vi "Control Panel.vi"(8 "error in (no error)":errorcluster, 11 "Power Supply.lvclass":refnum<class "Power Supply.lvclass">) -> (0 "error out":errorcluster, 3 "Power Supply.lvclass out":refnum<class "Power Supply.lvclass">)   [LabVIEW 2017, in "Power Supply.lvclass"]
uses:
  Power Supply.lvclass
  Utility Classes/InstrPtr/InstrPtr.lvclass
  Magnet status.ctl
  Power Supply.lvclass/Power Supply.ctl
  Global/Relative Sound Files.vi
  File IO/File IO.lvclass
panel:
  out "Was at persistent?":bool
  in  "Return to persistent?":bool
  out "log counter":dbl
  out "Going to Field?":bool
  out "Current Field":dbl[unit]
  out "Update UI":bool
  out "Status":T1
  out "*ips120":T2
  in  "Abort Field Sweep":bool
  out "done?":bool
  out "ILM Shut Down?":bool
  out "SH On":bool caption="Switch Heater"
  out "Persistent Mode":bool
  in  "SHcontrol":bool caption="Switch Heater"
  in  "gotopersistent":bool
  out "active":bool
  in  "Train\nMagnet":bool
  out "Busy":bool
  out "ready?":bool
  in  "rate":dbl[unit]=0.016666666666666666 caption="Rate" min=0.0 max=0.25
  in  "Goto":dbl[unit]
  in  "Clamp":bool
  in  "Check for Magnet":bool
  in  "Hold":bool
  in  "Goto Zero":bool
  in  "Goto Field":bool
  in  "endprgm":bool
  # "Magnet Control Panel"
  # "(at current field)"
  # "Off"
  # "On"
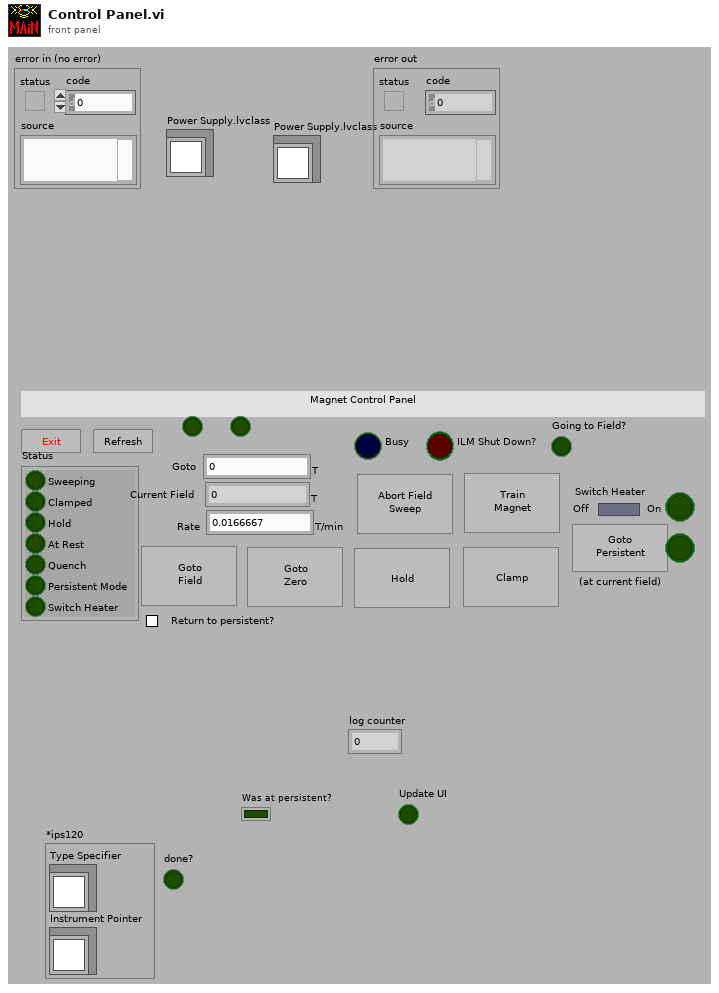
[diagram p1: front panel]
types:
  T1 = typedef "Power Supply.lvclass/Magnet status.ctl" = cluster{"Sweeping":bool, "Clamped":bool, "Hold":bool, "At Rest":bool, "Quench":bool, "Persistent Mode":bool, "Switch Heater":bool}
  T2 = cluster{"Type Specifier":refnum<class "Power Supply.lvclass">, "Instrument Pointer":refnum<class "InstrPtr.lvclass">}
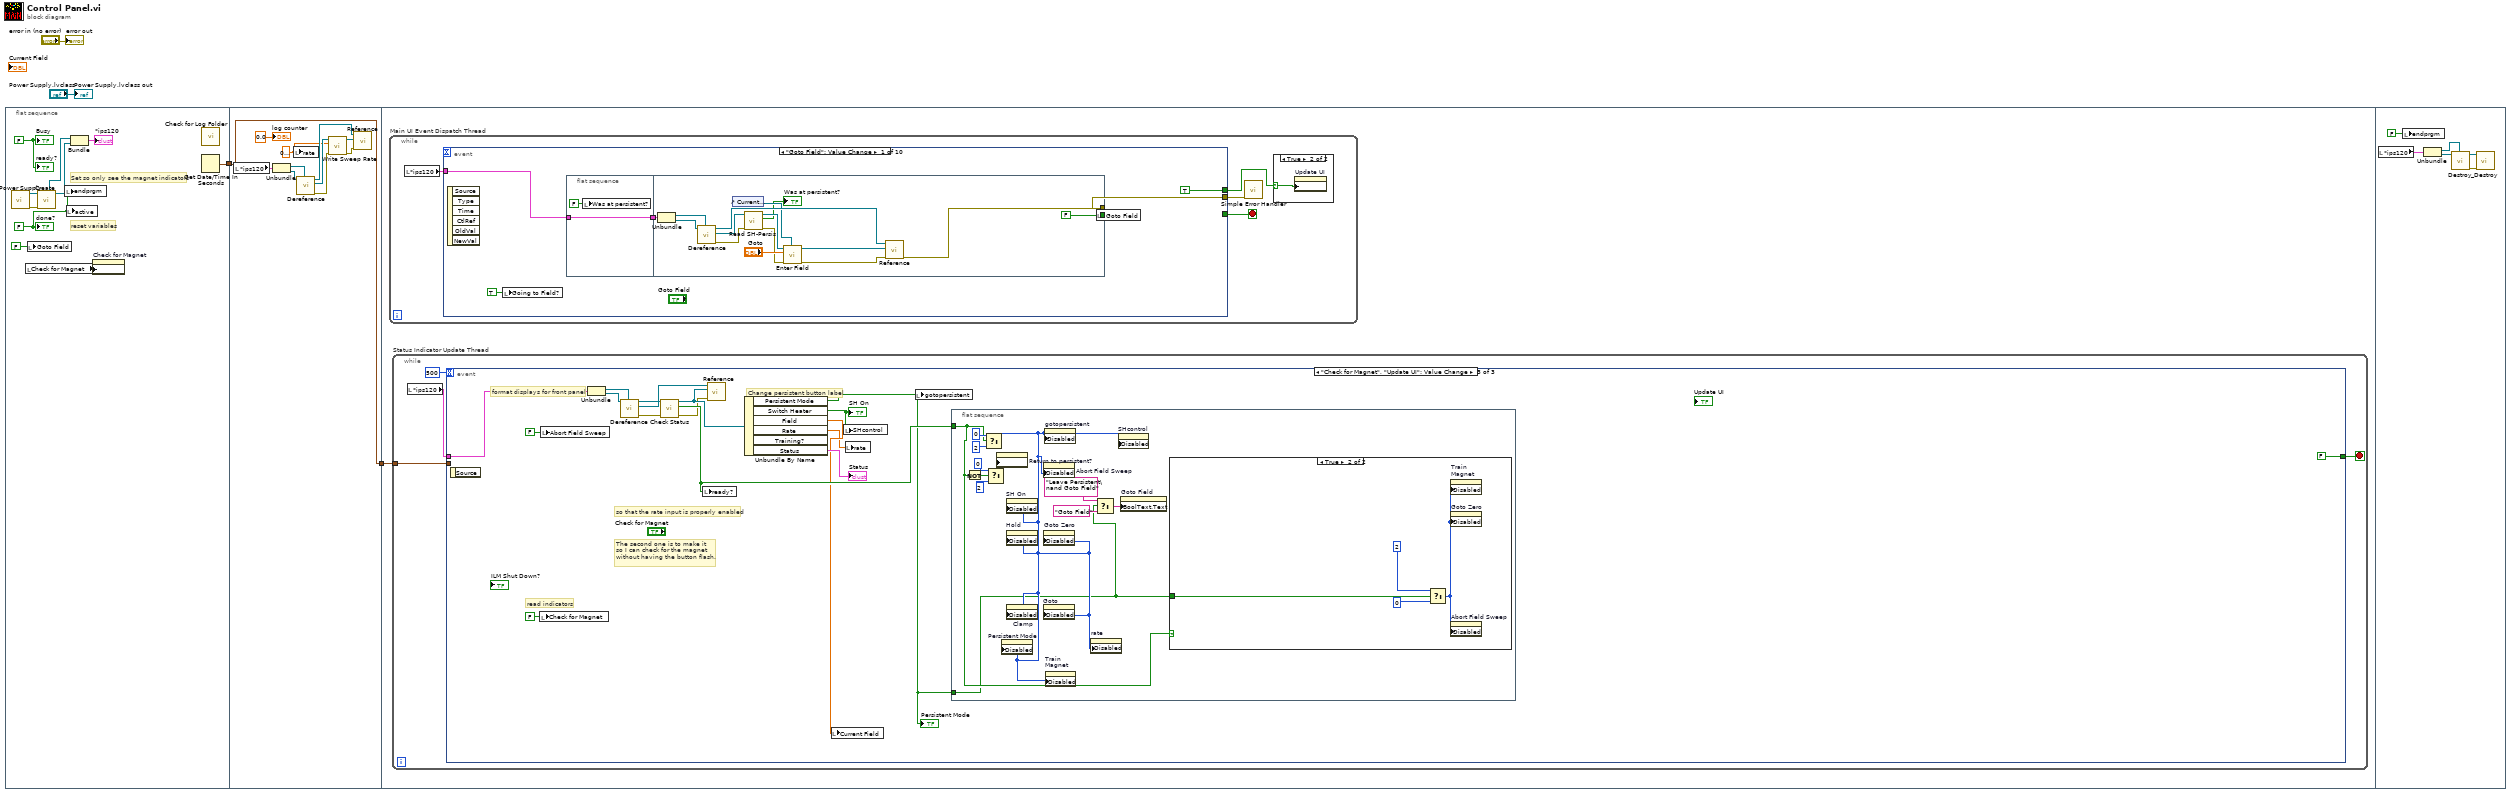
[diagram p0: block diagram]
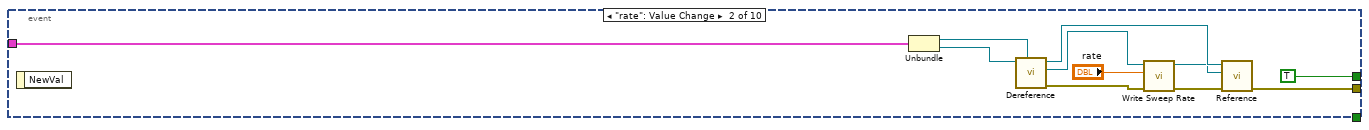
[diagram p3: hidden frame]
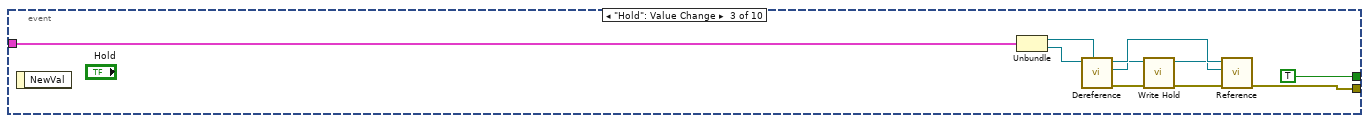
[diagram p4: hidden frame]
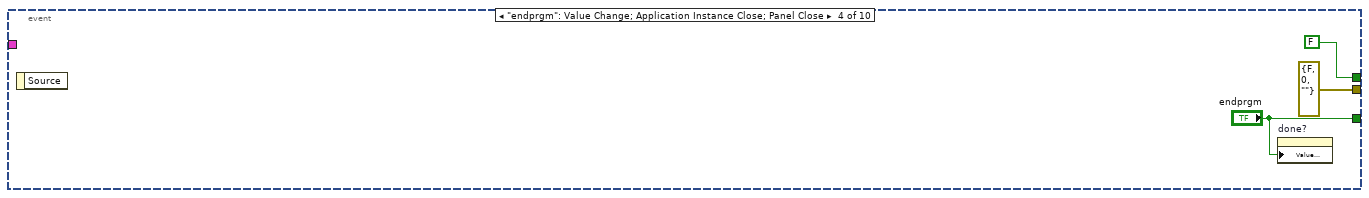
[diagram p5: hidden frame]
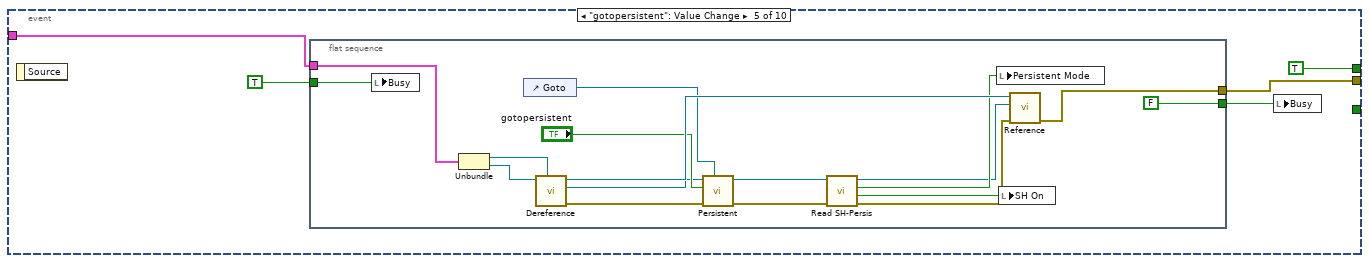
[diagram p6: hidden frame]
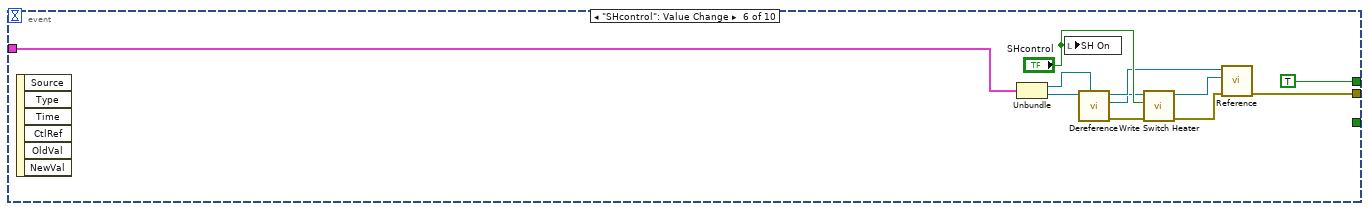
[diagram p7: hidden frame]
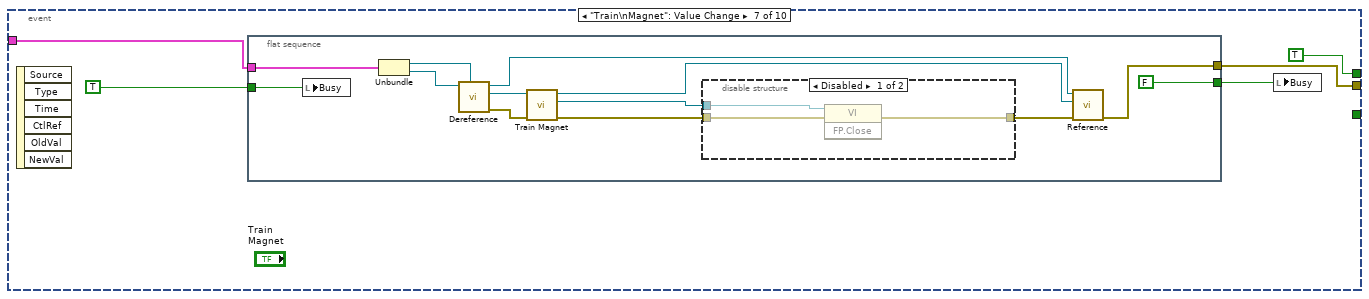
[diagram p8: hidden frame]
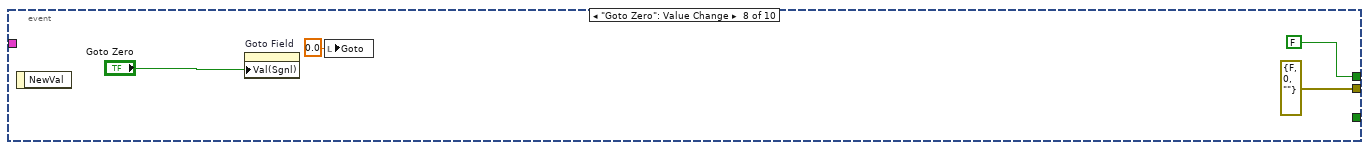
[diagram p10: hidden frame]
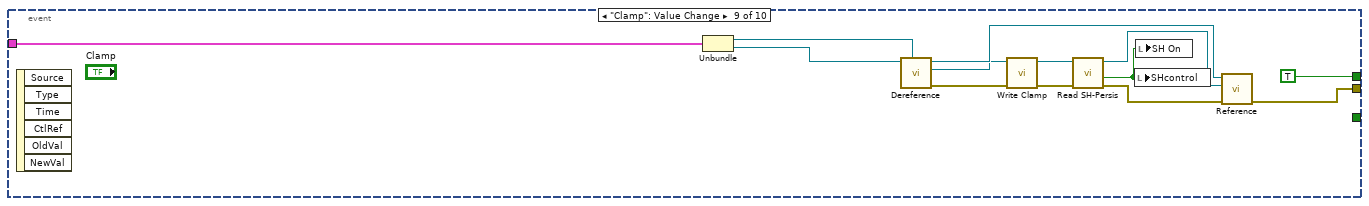
[diagram p11: hidden frame]
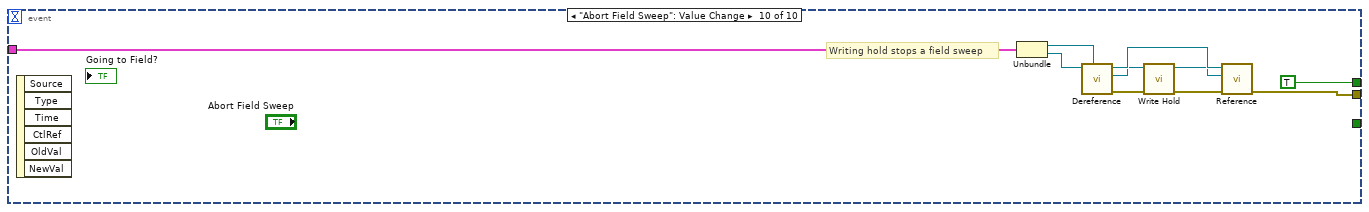
[diagram p12: hidden frame]
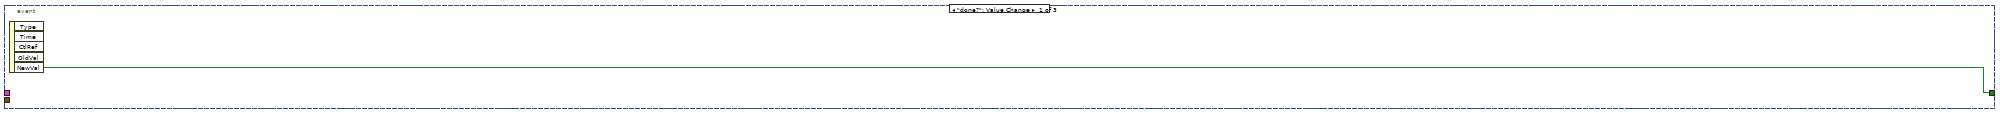
[diagram p13: hidden frame]
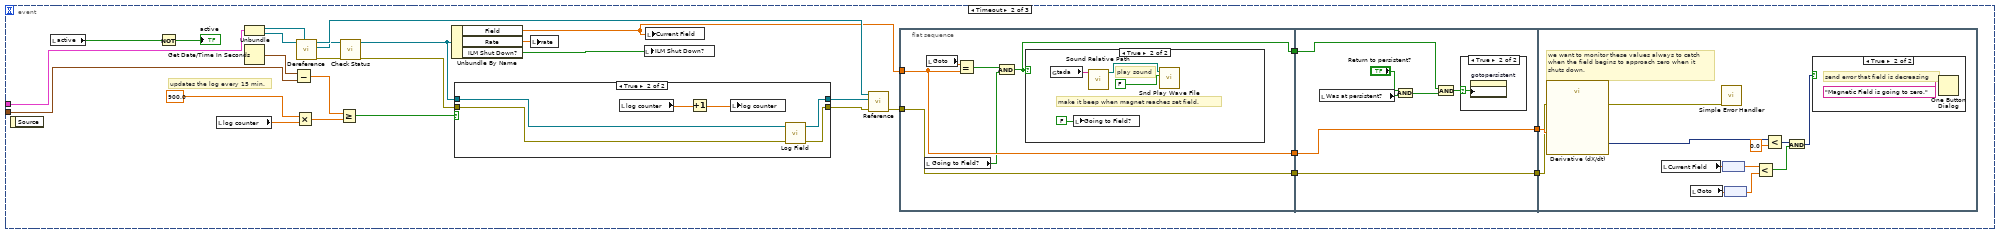
[diagram p14: hidden frame]
diagram:
  n1 = flat-sequence {
    tunnel: [w5] -> w2
    tunnel: w2 -> [w16]
    tunnel: [w16] -> w1
    tunnel: w1 -> [w26]
    frame #0 {
      w14 = FALSE
      w12 = FALSE
      # "Set so only see the magnet indicators"
      # "reset variables"
      n2 = call "Power Supply.vi"() -> ("error out"=w7:errorcluster, "Power Supply out"=w11:refnum<class "Power Supply.lvclass">)  [unwired: 10 in]
      n3 = local read "Check for Magnet"() -> (w13:bool)
      n4 = local write "Goto Field"(FALSE ("active")) -> ()
      n5 = call "Create.vi"("error in (no error)"=w7, "Instrument in"=w11) -> ("Instrument Pointer"=w10:refnum<class "InstrPtr.lvclass">, "Type Specifier"=w9:refnum<class "Power Supply.lvclass">)  [unwired: 7 in, 1 out]
      n6 = local write "endprgm"(w12) -> ()
      n7 = local write "active"(w12) -> ()
      n8 = Bundle("Type Specifier"=w9, "Instrument Pointer"=w10) -> (→"*ips120":T2)  [unwired: 1 in]
      n9 = property on="Check for Magnet" class="Bool (strict)"("Value (Signaling)"=w13) -> ()  [unwired: 2 in, 2 out]
      n10 = call "Check for Log Folder.vi"() -> ()  [unwired: 1 out]
      n11 = Get Date/Time In Seconds() -> (seconds since 1Jan1904=w5:timestamp)
      "ready?" <- w14
      "Busy" <- w14
      "done?" <- w12
    }
    frame #1 {
      w17 = dbl[unit] 0.016666666666666666 ("rate")
      n12 = local read "*ips120"() -> (w18:T2)
      n13 = Unbundle(w18) -> ("Type Specifier"=w19:refnum<class "Power Supply.lvclass">, "Instrument Pointer"=w20:refnum<class "InstrPtr.lvclass">)
      n14 = local write "rate"(w17) -> ()
      n15 = call "Dereference.vi"("Type Specifier"=w19, "InstrPtr"=w20) -> ("error out"=w24:errorcluster, "Instrument out"=w23:refnum<class "Power Supply.lvclass">, "InstrPtr out"=w21:refnum<class "InstrPtr.lvclass">)  [unwired: 7 in]
      n16 = call-dynamic "Write Sweep Rate.vi"("error in (no error)"=w24, "rate"=w17, "Power Supply in"=w23) -> ("error out"=w25:errorcluster, "Power Supply out"=w22:refnum<class "Power Supply.lvclass">)  [unwired: 7 in]
      n17 = call "Reference.vi"("error in (no error)"=w25, "Instrument"=w22, "InstrPtr in"=w21) -> ()  [unwired: 8 in, 1 out]
      "log counter" <- 0.0 ("log counter")
    }
    frame #2 {
      n18 = while "Main UI Event Dispatch Thread" {
        stop <- w29 stop-if-true
        n19 = local read "*ips120"() -> (w27:T2)
        n20 = event shown="[0] \"Goto Field\": Value Change" {
          selector: _ -> [_ _ _ _ _ _ _ _ _ _]
          dyn-events: _ -> [_ _ _ _ _ _ _ _ _ _]
          timeout: _ -> [_ _ _ _ _ _ _ _ _ _]
          tunnel: [_ _ _ "endprgm" _ _ _ _ _ _] -> w29
          tunnel: w27 -> [w37 w65 w75 _ w83 w110 w116 _ w143 w152]
          tunnel: [w35 w56 w74 errorcluster {"status"=FALSE, "code"=0, "source"=""} ("error out") w82 w104 w115 errorcluster {"status"=FALSE, "code"=0, "source"=""} ("error out") w139 w153] -> w30
          tunnel: [TRUE TRUE TRUE FALSE TRUE TRUE TRUE FALSE TRUE TRUE] -> w28
          event "Goto Field": Value Change {
            n21 = event-data() -> ()  [unwired: 7 out]
            n22 = local write "Going to Field?"(TRUE ("Going to Field?")) -> ()
            n23 = flat-sequence {
              tunnel: w37 -> [w39]
              tunnel: [w39] -> w32
              tunnel: [FALSE ("Goto Field")] -> w36
              tunnel: [w47] -> w35
              tunnel: w32 -> [w52]
              frame #0 {
                n24 = local write "Was at persistent?"(FALSE ("Was at persistent?")) -> ()
              }
              frame #1 {
                n25 = Unbundle(w52) -> ("Type Specifier"=w54:refnum<class "Power Supply.lvclass">, "Instrument Pointer"=w53:refnum<class "InstrPtr.lvclass">)
                n26 = call "Dereference.vi"("Type Specifier"=w54, "InstrPtr"=w53) -> ("error out"=w42:errorcluster, "Instrument out"=w44:refnum<class "Power Supply.lvclass">, "InstrPtr out"=w51:refnum<class "InstrPtr.lvclass">)  [unwired: 7 in]
                n27 = control-ref of="Current Field"() -> (w46:refnum<vi>)
                n28 = call-dynamic "Read SH-Persis.vi"("error in (no error)"=w42, "Power Supply in"=w44) -> ("error out"=w41:errorcluster, "pers?"=→"Was at persistent?":bool, "Power Supply out"=w43:refnum<class "Power Supply.lvclass">)  [unwired: 4 in, 3 out]
                n29 = call-dynamic "Enter Field.vi"("Field monitor"=w46, "error in (no error)"=w41, "Target field"="Goto", "Power Supply in"=w43) -> ("error out"=w49:errorcluster, "Power Supply out"=w50:refnum<class "Power Supply.lvclass">)  [unwired: 6 in]
                n30 = call "Reference.vi"("error in (no error)"=w49, "Instrument"=w50, "InstrPtr in"=w51) -> ("error out"=w47:errorcluster)  [unwired: 8 in]
              }
            }
            n31 = local write "Goto Field"(w36) -> ()
          }
          event "rate": Value Change {
            n32 = event-data() -> ()  [unwired: 2 out]
            n33 = Unbundle(w65) -> ("Type Specifier"=w64:refnum<class "Power Supply.lvclass">, "Instrument Pointer"=w63:refnum<class "InstrPtr.lvclass">)
            n34 = call "Dereference.vi"("Type Specifier"=w64, "InstrPtr"=w63) -> ("error out"=w58:errorcluster, "Instrument out"=w60:refnum<class "Power Supply.lvclass">, "InstrPtr out"=w62:refnum<class "InstrPtr.lvclass">)  [unwired: 7 in]
            n35 = call-dynamic "Write Sweep Rate.vi"("error in (no error)"=w58, "rate"="rate", "Power Supply in"=w60) -> ("error out"=w57:errorcluster, "Power Supply out"=w61:refnum<class "Power Supply.lvclass">)  [unwired: 7 in]
            n36 = call "Reference.vi"("error in (no error)"=w57, "Instrument"=w61, "InstrPtr in"=w62) -> ("error out"=w56:errorcluster)  [unwired: 8 in]
          }
          event "Hold": Value Change {
            n37 = event-data() -> ()  [unwired: 2 out]
            n38 = Unbundle(w75) -> ("Type Specifier"=w72:refnum<class "Power Supply.lvclass">, "Instrument Pointer"=w73:refnum<class "InstrPtr.lvclass">)
            n39 = call "Dereference.vi"("Type Specifier"=w72, "InstrPtr"=w73) -> ("error out"=w67:errorcluster, "Instrument out"=w70:refnum<class "Power Supply.lvclass">, "InstrPtr out"=w71:refnum<class "InstrPtr.lvclass">)  [unwired: 7 in]
            n40 = call-dynamic "Write Hold.vi"("error in (no error)"=w67, "Power Supply in"=w70) -> ("error out"=w68:errorcluster, "Power Supply out"=w69:refnum<class "Power Supply.lvclass">)  [unwired: 8 in]
            n41 = call "Reference.vi"("error in (no error)"=w68, "Instrument"=w69, "InstrPtr in"=w71) -> ("error out"=w74:errorcluster)  [unwired: 8 in]
          }
          event "endprgm": Value Change; Application Instance Close; Panel Close {
            n42 = event-data() -> ()  [unwired: 2 out]
            n43 = property on="done?" class="Bool (strict)"("Value (Signaling)"="endprgm") -> ()  [unwired: 2 in, 2 out]
          }
          event "gotopersistent": Value Change {
            n44 = event-data() -> ()  [unwired: 2 out]
            n45 = flat-sequence {
              tunnel: w83 -> [w100]
              tunnel: [w99] -> w82
              tunnel: TRUE -> [w85]
              tunnel: [FALSE] -> w79
              frame #0 {
                n46 = local write "Busy"(w85) -> ()
                n47 = Unbundle(w100) -> ("Type Specifier"=w93:refnum<class "Power Supply.lvclass">, "Instrument Pointer"=w92:refnum<class "InstrPtr.lvclass">)
                n48 = control-ref of="Goto"() -> (w95:refnum<vi>)
                n49 = call "Dereference.vi"("Type Specifier"=w93, "InstrPtr"=w92) -> ("error out"=w90:errorcluster, "Instrument out"=w91:refnum<class "Power Supply.lvclass">, "InstrPtr out"=w96:refnum<class "InstrPtr.lvclass">)  [unwired: 7 in]
                n50 = call-dynamic "Persistent.vi"("Field monitor ref"=w95, "error in (no error)"=w90, "Go to persistent mode?"="gotopersistent", "Power Supply in"=w91) -> ("error out"=w98:errorcluster, "Power Supply out"=w97:refnum<class "Power Supply.lvclass">)  [unwired: 6 in]
                n51 = call-dynamic "Read SH-Persis.vi"("error in (no error)"=w98, "Power Supply in"=w97) -> ("error out"=w86:errorcluster, "SHon?"=w88:bool, "pers?"=w89:bool, "Power Supply out"=w87:refnum<class "Power Supply.lvclass">)  [unwired: 4 in, 2 out]
                n52 = local write "Persistent Mode"(w89) -> ()
                n53 = local write "SH On"(w88) -> ()
                n54 = call "Reference.vi"("error in (no error)"=w86, "Instrument"=w87, "InstrPtr in"=w96) -> ("error out"=w99:errorcluster)  [unwired: 8 in]
              }
            }
            n55 = local write "Busy"(w79) -> ()
          }
          event "SHcontrol": Value Change {
            n56 = event-data() -> ()  [unwired: 7 out]
            n57 = Unbundle(w110) -> ("Type Specifier"=w108:refnum<class "Power Supply.lvclass">, "Instrument Pointer"=w109:refnum<class "InstrPtr.lvclass">)
            n58 = local write "SH On"("SHcontrol") -> ()
            n59 = call "Dereference.vi"("Type Specifier"=w108, "InstrPtr"=w109) -> ("error out"=w103:errorcluster, "Instrument out"=w102:refnum<class "Power Supply.lvclass">, "InstrPtr out"=w107:refnum<class "InstrPtr.lvclass">)  [unwired: 7 in]
            n60 = call-dynamic "Write Switch Heater.vi"("error in (no error)"=w103, "Turn SH On?"="SHcontrol", "Power Supply in"=w102) -> ("error out"=w105:errorcluster, "Power Supply out"=w106:refnum<class "Power Supply.lvclass">)  [unwired: 7 in]
            n61 = call "Reference.vi"("error in (no error)"=w105, "Instrument"=w106, "InstrPtr in"=w107) -> ("error out"=w104:errorcluster)  [unwired: 8 in]
          }
          event "Train\nMagnet": Value Change {
            n62 = event-data() -> ()  [unwired: 7 out]
            n63 = flat-sequence {
              tunnel: w116 -> [w129]
              tunnel: [w125] -> w115
              tunnel: [FALSE] -> w113
              tunnel: TRUE -> [w120]
              frame #0 {
                n64 = local write "Busy"(w120) -> ()
                n65 = Unbundle(w129) -> ("Type Specifier"=w128:refnum<class "Power Supply.lvclass">, "Instrument Pointer"=w127:refnum<class "InstrPtr.lvclass">)
                n66 = call "Dereference.vi"("Type Specifier"=w128, "InstrPtr"=w127) -> ("error out"=w123:errorcluster, "Instrument out"=w124:refnum<class "Power Supply.lvclass">, "InstrPtr out"=w126:refnum<class "InstrPtr.lvclass">)  [unwired: 7 in]
                n67 = call-dynamic "Train Magnet.vi"("error in (no error)"=w123, "Power Supply in"=w124) -> ("error out"=w118:errorcluster, "This VI"=w119:refnum<vi>, "Power Supply out"=w122:refnum<class "Power Supply.lvclass">)  [unwired: 7 in]
                n68 = disable-structure shown="Disabled" {
                  disable-tunnel: w119 -> [w132 _]
                  disable-tunnel: w118 -> [w131 w133]
                  disable-tunnel: [w130 w133] -> w117
                  frame Disabled {
                    n69 = invoke class="VI" method="FP.Close"(reference=w132, error in=w131) -> (error out=w130:errorcluster)  [unwired: 1 in, 2 out]
                  }
                  frame Enabled {
                  }
                }
                n70 = call "Reference.vi"("error in (no error)"=w117, "Instrument"=w122, "InstrPtr in"=w126) -> ("error out"=w125:errorcluster)  [unwired: 8 in]
              }
            }
            n71 = local write "Busy"(w113) -> ()
          }
          event "Goto Zero": Value Change {
            n72 = event-data() -> ()  [unwired: 2 out]
            n73 = property on="Goto Field" class="Bool (strict)"("Val(Sgnl)"="Goto Zero") -> ()  [unwired: 2 in, 2 out]
            n74 = local write "Goto"(dbl[unit] 0.0 ("Goto")) -> ()
          }
          event "Clamp": Value Change {
            n75 = event-data() -> ()  [unwired: 7 out]
            n76 = Unbundle(w143) -> ("Type Specifier"=w147:refnum<class "Power Supply.lvclass">, "Instrument Pointer"=w146:refnum<class "InstrPtr.lvclass">)
            n77 = call "Dereference.vi"("Type Specifier"=w147, "InstrPtr"=w146) -> ("error out"=w142:errorcluster, "Instrument out"=w144:refnum<class "Power Supply.lvclass">, "InstrPtr out"=w145:refnum<class "InstrPtr.lvclass">)  [unwired: 7 in]
            n78 = call-dynamic "Write Clamp.vi"("error in (no error)"=w142, "Power Supply in"=w144) -> ("error out"=w149:errorcluster, "Power Supply out"=w150:refnum<class "Power Supply.lvclass">)  [unwired: 8 in]
            n79 = call-dynamic "Read SH-Persis.vi"("error in (no error)"=w149, "Power Supply in"=w150) -> ("error out"=w141:errorcluster, "SHon?"=w148:bool, "Power Supply out"=w140:refnum<class "Power Supply.lvclass">)  [unwired: 4 in, 3 out]
            n80 = local write "SHcontrol"(w148) -> ()
            n81 = local write "SH On"(w148) -> ()
            n82 = call "Reference.vi"("error in (no error)"=w141, "Instrument"=w140, "InstrPtr in"=w145) -> ("error out"=w139:errorcluster)  [unwired: 8 in]
          }
          event "Abort Field Sweep": Value Change {
            # "Writing hold stops a field sweep"
            n83 = event-data() -> ()  [unwired: 7 out]
            n84 = Unbundle(w152) -> ("Type Specifier"=w160:refnum<class "Power Supply.lvclass">, "Instrument Pointer"=w159:refnum<class "InstrPtr.lvclass">)
            n85 = call "Dereference.vi"("Type Specifier"=w160, "InstrPtr"=w159) -> ("error out"=w157:errorcluster, "Instrument out"=w154:refnum<class "Power Supply.lvclass">, "InstrPtr out"=w158:refnum<class "InstrPtr.lvclass">)  [unwired: 7 in]
            n86 = call-dynamic "Write Hold.vi"("error in (no error)"=w157, "Power Supply in"=w154) -> ("error out"=w156:errorcluster, "Power Supply out"=w155:refnum<class "Power Supply.lvclass">)  [unwired: 8 in]
            n87 = call "Reference.vi"("error in (no error)"=w156, "Instrument"=w155, "InstrPtr in"=w158) -> ("error out"=w153:errorcluster)  [unwired: 8 in]
          }
        }
        n88 = call <vilib>:"Simple Error Handler.vi"("error in (no error)"=w30) -> ()  [unwired: 4 in, 5 out]
        n89 = case shown="True" w28 {
          selector: w28 -> [_ w31]
          frame False {
          }
          frame True {
            n90 = property on="Update UI" class="Bool (strict)"("Value (Signaling)"=w31) -> ()  [unwired: 2 in, 2 out]
          }
        }
      }
      n91 = while "Status Indicator Update Thread" {
        tunnel: w26 -> [w161]
        stop <- w163 stop-if-true
        n92 = local read "*ips120"() -> (w162:T2)
        n93 = event shown="[2] \"Check for Magnet\", \"Update UI\": Value Change" {
          selector: _ -> [_ _ _]
          dyn-events: _ -> [_ _ _]
          timeout: 500 -> [_ _ _]
          tunnel: [w165 _ FALSE] -> w163
          tunnel: w162 -> [_ w191 w239]
          tunnel: w161 -> [_ w190 _]
          event "done?": Value Change {
            n94 = event-data() -> ("NewVal"=w165:bool)  [unwired: 5 out]
          }
          event Timeout {
            # "updates the log every 15 min."
            n95 = event-data() -> ()  [unwired: 2 out]
            n96 = local read "active"() -> (w193:bool)
            n97 = Not(x=w193) -> (.not. x?=→"active":bool)
            n98 = local read "log counter"() -> (w173:dbl)
            n99 = Unbundle(w191) -> ("Type Specifier"=w186:refnum<class "Power Supply.lvclass">, "Instrument Pointer"=w187:refnum<class "InstrPtr.lvclass">)
            n100 = Get Date/Time In Seconds() -> (seconds since 1Jan1904=w176:timestamp)
            n101 = Subtract(x=w176, y=w190) -> (x-y=w171:dbl)
            n102 = Multiply(x=900.0 ("millisecond multiple"), y=w173) -> (x*y=w172:dbl)
            n103 = call "Dereference.vi"("Type Specifier"=w186, "InstrPtr"=w187) -> ("error out"=w185:errorcluster, "Instrument out"=w184:refnum<class "Power Supply.lvclass">, "InstrPtr out"=w188:refnum<class "InstrPtr.lvclass">)  [unwired: 7 in]
            n104 = Greater Or Equal?(x=w171, y=w172) -> (x >= y?=w177:bool)
            n105 = call-dynamic "Check Status.vi"("error in (no error)"=w185, "Power Supply in"=w184) -> ("error out"=w178:errorcluster, "Power Supply out"=w179:refnum<class "Power Supply.lvclass">)  [unwired: 6 in, 2 out]
            n106 = Unbundle By Name(w179) -> ("Field"=w183:dbl[unit], "Rate"=w175:dbl[unit], "ILM Shut Down?"=w189:bool)
            n107 = case shown="True" w177 {
              tunnel: [w226 w232] -> w181
              tunnel: [w225 w231] -> w180
              tunnel: w179 -> [w226 w230]
              tunnel: w178 -> [w225 w229]
              frame False {
              }
              frame True {
                n108 = local read "log counter"() -> (w228:dbl)
                n109 = Increment(x=w228) -> (x+1=w227:dbl)
                n110 = local write "log counter"(w227) -> ()
                n111 = call "Log Field.vi"("error in (no error)"=w229, "Power Supply In"=w230) -> ("error out"=w231:errorcluster, "Power Supply Out"=w232:refnum<class "Power Supply.lvclass">)  [unwired: 8 in]
              }
            }
            n112 = local write "rate"(w175) -> ()
            n113 = local write "ILM Shut Down?"(w189) -> ()
            n114 = local write "Current Field"(w183) -> ()
            n115 = call "Reference.vi"("error in (no error)"=w180, "Instrument"=w181, "InstrPtr in"=w188) -> ("error out"=w182:errorcluster)  [unwired: 8 in]
            n116 = flat-sequence {
              tunnel: w182 -> [w199]
              tunnel: w183 -> [w197]
              tunnel: [w197] -> w170
              tunnel: [w199] -> w169
              tunnel: [w194] -> w168
              tunnel: w170 -> [w210]
              tunnel: [w210] -> w167
              tunnel: w169 -> [w209]
              tunnel: [w209] -> w166
              tunnel: w168 -> [w207]
              tunnel: w167 -> [w223]
              tunnel: w166 -> [w222]
              frame #0 {
                n117 = local read "Going to Field?"() -> (w195:bool)
                n118 = local read "Goto"() -> (w198:dbl[unit])
                n119 = Equal?(x=w198, y=w197) -> (x = y?=w196:bool)
                n120 = And(x=w196, y=w195) -> (x .and. y?=w194:bool)
                n121 = case shown="True" w194 {
                  frame False {
                  }
                  frame True {
                    # "make it beep when magnet reaches set field."
                    # "play sound"
                    n122 = global read "Relative Sound Files.vi" "tada"() -> (w201:string)
                    n123 = local write "Going to Field?"(FALSE ("Going to Field?")) -> ()
                    n124 = call "Sound Relative Path.vi"("Sound"=w201) -> ("Relative Path"=w202:path)  [unwired: 10 in]
                    n125 = call <vilib>:"Snd Play Wave File.vi"("wait until finish (T)"=FALSE, "wave file path"=w202) -> ()  [unwired: 1 in, 9 out]
                  }
                }
              }
              frame #1 {
                n126 = local read "Was at persistent?"() -> (w206:bool)
                n127 = And(x="Return to persistent?", y=w206) -> (x .and. y?=w204:bool)
                n128 = And(x=w207, y=w204) -> (x .and. y?=w208:bool)
                n129 = case shown="True" w208 {
                  selector: w208 -> [_ w211]
                  frame False {
                  }
                  frame True {
                    n130 = property on="gotopersistent" class="Bool (strict)"("Value (Signaling)"=w211) -> ()  [unwired: 2 in, 2 out]
                  }
                }
              }
              frame #2 {
                # "we want to monitor these values always to catch\nwhen the field begins to approach zero when it\nshuts down."
                n131 = call "Derivative (dX/dt)"("error in (no error)"=w222, "Signals"=w223) -> ("error out"=w217:errorcluster, "Result"=w221:dynamicdata)  [unwired: 4 out]
                n132 = local read "Current Field"() -> (w213:dbl[unit])
                n133 = local read "Goto"() -> (w215:dbl[unit])
                n134 = call <vilib>:"Simple Error Handler.vi"("error in (no error)"=w217) -> ()  [unwired: 4 in, 5 out]
                n135 = node(w213) -> (w212:dbl)
                n136 = node(w215) -> (w214:dbl)
                n137 = Less?(x=w212, y=w214) -> (x < y?=w216:bool)
                n138 = Less?(x=w221, y=0.0) -> (x < y?=w219:dynamicdata)
                n139 = And(x=w219, y=w216) -> (x .and. y?=w218:dynamicdata)
                n140 = case shown="True" w218 {
                  frame False {
                  }
                  frame True {
                    # "send error that field is decreasing"
                    n141 = One Button Dialog(message="Magnetic Field is going to zero.") -> ()  [unwired: 1 in, 1 out]
                  }
                }
              }
            }
          }
          event "Check for Magnet", "Update UI": Value Change {
            # "format displays for front panel"
            # "read indicators"
            # "so that the rate input is properly enabled"
            # "Change persistent button label"
            # "The second one is to make it\nso I can check for the magnet\nwithout having the button flash."
            n142 = event-data() -> ()  [unwired: 2 out]
            n143 = local write "Check for Magnet"(FALSE) -> ()
            n144 = local write "Abort Field Sweep"(FALSE ("Abort Field Sweep")) -> ()
            n145 = Unbundle(w239) -> ("Type Specifier"=w240:refnum<class "Power Supply.lvclass">, "Instrument Pointer"=w245:refnum<class "InstrPtr.lvclass">)
            n146 = call "Dereference.vi"("Type Specifier"=w240, "InstrPtr"=w245) -> ("error out"=w244:errorcluster, "Instrument out"=w243:refnum<class "Power Supply.lvclass">, "InstrPtr out"=w241:refnum<class "InstrPtr.lvclass">)  [unwired: 7 in]
            n147 = call-dynamic "Check Status.vi"("error in (no error)"=w244, "Power Supply in"=w243) -> ("error out"=w238:errorcluster, "Ready?"=w247:bool, "Power Supply out"=w242:refnum<class "Power Supply.lvclass">)  [unwired: 6 in, 1 out]
            n148 = local write "ready?"(w247) -> ()
            n149 = call "Reference.vi"("error in (no error)"=w238, "Instrument"=w242, "InstrPtr in"=w241) -> ()  [unwired: 8 in, 1 out]
            n150 = Unbundle By Name(w242) -> ("Persistent Mode"=w235:bool, "Switch Heater"=w246:bool, "Field"=w236:dbl[unit], "Rate"=w233:dbl[unit], "Status"=→"Status":T1)  [unwired: 1 out]
            "Persistent Mode" <- w235
            "SH On" <- w246
            n151 = local write "Current Field"(w236) -> ()
            n152 = local write "SHcontrol"(w246) -> ()
            n153 = local write "rate"(w233) -> ()
            n154 = local write "gotopersistent"(w235) -> ()
            n155 = flat-sequence {
              tunnel: w235 -> [w250]
              tunnel: w247 -> [w256]
              frame #0 {
                n156 = Not(x=w256) -> (.not. x?=w255:bool)
                n157 = Select(t=0, s=w256, f=2) -> (s? t:f=w259:i32)
                n158 = Select(t=0, s=w255, f=2) -> (s? t:f=w254:i32)
                n159 = property on="Return to persistent?" class="Bool (strict)"("DisabledEnum"=w254) -> ()  [unwired: 2 in, 2 out]
                n160 = property on="Persistent Mode" class="Bool (strict)"("Disabled"=w259) -> ()  [unwired: 2 in, 2 out]
                n161 = property on="SH On" class="Bool (strict)"("Disabled"=w259) -> ()  [unwired: 2 in, 2 out]
                n162 = property on="Hold" class="Bool"("Disabled"=w259) -> ()  [unwired: 2 in, 2 out]
                n163 = property on="Clamp" class="Bool"("Disabled"=w259) -> ()  [unwired: 2 in, 2 out]
                n164 = property on="Abort Field Sweep" class="Bool (strict)"("Disabled"=w259) -> ()  [unwired: 2 in, 2 out]
                n165 = property on="Goto Zero" class="Bool"("Disabled"=w259) -> ()  [unwired: 2 in, 2 out]
                n166 = property on="Goto" class="DigNum (strict)"("Disabled"=w259) -> ()  [unwired: 2 in, 2 out]
                n167 = property on="gotopersistent" class="Bool (strict)"("Disabled"=w259) -> ()  [unwired: 2 in, 2 out]
                n168 = property on="Train\nMagnet" class="Bool"("Disabled"=w259) -> ()  [unwired: 2 in, 2 out]
                n169 = property on="rate" class="DigNum (strict)"("Disabled"=w259) -> ()  [unwired: 2 in, 2 out]
                n170 = Select(t="Leave Persistent\nand Goto Field", s=w250, f="Goto Field") -> (s? t:f=w252:string)
                n171 = property on="SHcontrol" class="Bool (strict)"("Disabled"=w259) -> ()  [unwired: 2 in, 2 out]
                n172 = property on="Goto Field" class="Bool (strict)"("BoolText.Text"=w252) -> ()  [unwired: 2 in, 2 out]
                n173 = case shown="True" w256 {
                  tunnel: w250 -> [_ w263]
                  frame False {
                  }
                  frame True {
                    n174 = Select(t=2, s=w263, f=0) -> (s? t:f=w262:i32)
                    n175 = property on="Train\nMagnet" class="Bool"("Disabled"=w262) -> ()  [unwired: 2 in, 2 out]
                    n176 = property on="Goto Zero" class="Bool"("Disabled"=w262) -> ()  [unwired: 2 in, 2 out]
                    n177 = property on="Abort Field Sweep" class="Bool (strict)"("Disabled"=w262) -> ()  [unwired: 2 in, 2 out]
                  }
                }
              }
            }
          }
        }
      }
    }
    frame #3 {
      n178 = local read "*ips120"() -> (w270:T2)
      n179 = local write "endprgm"(FALSE) -> ()
      n180 = Unbundle(w270) -> ("Type Specifier"=w267:refnum<class "Power Supply.lvclass">, "Instrument Pointer"=w269:refnum<class "InstrPtr.lvclass">)
      n181 = call "Destroy.vi"("Type Specifier"=w267, "InstrPtr in"=w269) -> ("error out"=w266:errorcluster, "final Instrument"=w268:refnum<class "Power Supply.lvclass">)  [unwired: 8 in]
      n182 = call-dynamic "_Destroy.vi"("error in (no error)"=w266, "Instrument in"=w268) -> ()  [unwired: 9 in, 1 out]
    }
  }
  "Power Supply.lvclass out" <- "Power Supply.lvclass"
  "error out" <- "error in (no error)"
